vi "Coherency_Cal.vi"() -> ()   [LabVIEW 2019]
panel:
  out "Fin_Coherent":dbl
  out "Bin_":dbl
  in  "Fsampling":dbl
  in  "Nsamples":dbl
  in  "Fin":dbl
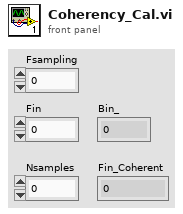
[diagram p1: front panel]
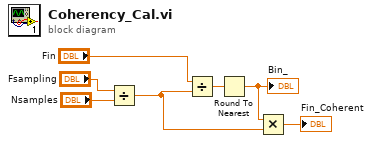
[diagram p0: block diagram]
diagram:
  n1 = Divide(x="Fsampling", y="Nsamples") -> (x/y=w2:dbl)
  n2 = Divide(x="Fin", y=w2) -> (x/y=w4:dbl)
  n3 = Round To Nearest(number=w4) -> (nearest integer value=w3:dbl)
  "Bin_" <- w3
  n4 = Multiply(x=w3, y=w2) -> (x*y=→"Fin_Coherent":dbl)
